vi "Column Separator.vi"() -> (0 "delimiter":string)   [LabVIEW 2020, in "Astemes_CSVReportPlugin.lvlib" / "TestStand Result Handler.lvclass"]
uses:
  TestStand Result Handler.lvclass
  TestStand Result Handler.lvclass/TestStand Result Handler.ctl
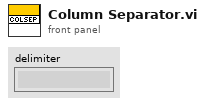
[diagram p1: front panel]
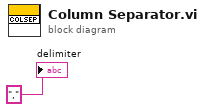
[diagram p0: block diagram]
diagram:
  "delimiter" <- "," ("delimiter")
